vi "buildClassMethodName.vi"(1 "methodName":string, 2 "classPath":path) -> (0 "methodName":string)   [LabVIEW 2023]
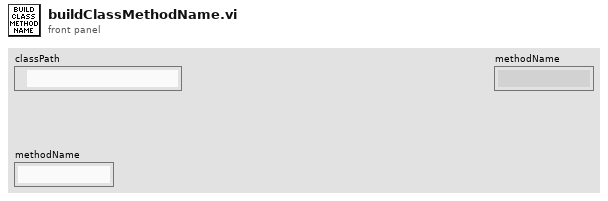
[diagram p1: front panel]
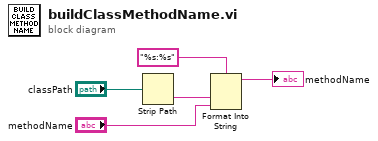
[diagram p0: block diagram]
diagram:
  n1 = Strip Path(path="classPath") -> (name=w2:string)  [unwired: 1 out]
  n2 = Format Into String(format string="%s:%s", w2, "methodName") -> (resulting string=→"methodName":string)  [unwired: 2 in, 1 out]
